vi "FindClusterCtlRefs.vi"(8 "error in (no error)":errorcluster, 10 "CLT Ref Array":refnum<vi>[](array[refnum]), 11 "CTL Name Array":string[](array[string])) -> (0 "error out":errorcluster, 2 "Cluster CTL Array":refnum<vi>[](array[refnum]), 3 "Cluster CTL Name Array":string[](array[string]))   [LabVIEW 2018, in "CtlReferences.lvlib" / "CtlReferences.lvclass"]
doc: "Get the refs of the CTLS in a Cluster.\nThis VI will also get the CTLS of any clusters inside the cluster... etc."
uses:
  CtlReferences.lvclass
  TypeDefs/ClassID_Enum.ctl
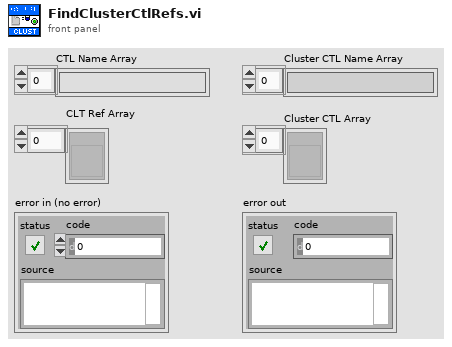
[diagram p1: front panel]
types:
  T1 = typedef "CtlReferences.lvlib/CtlReferences.lvclass/ClassID_Enum.ctl" = enum32{"0 <undefined>", "1 <undefined>", "2 <undefined>", "Generic", "Decoration", "Text", "Control", "ColorBox", "Boolean", "RefNum", "Variant", "Path", "ListBox", "Table", "Array", "Picture", "ActiveXContainer", "Numeric", "Digital", "NamedNumeric", "ColorRamp", "Slide", "GraphOrChart", "WaveformChart", "WaveformGraph", "IntensityChart", "IntensityGraph", "String", "IOName", "ComboBox", "Cluster", "Panel", "Knob", "NumWithScale", "Ring", "Enum", "GObject", "Plot", "Cursor", "NumericText", "Scale", "ColorScale", "GraphScale", "ColorGraphScale", "TypedRefNum", "OldKnobScale", "MCListbox", "MeasureData", "BVTag", "DAQName", "VISAName", "IVIName", "SlideScale", "TabControl", "Page", "TabArrayTabControl", "ConPane"}
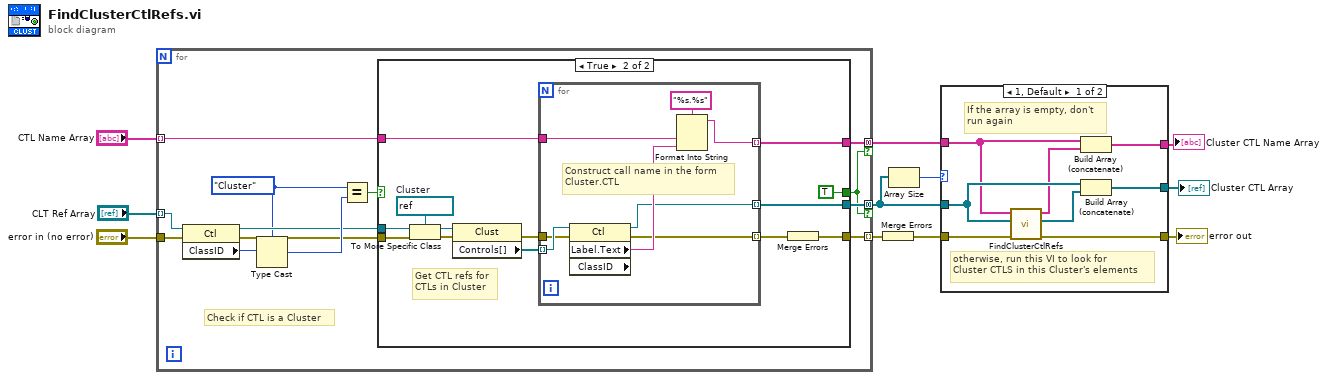
[diagram p0: block diagram]
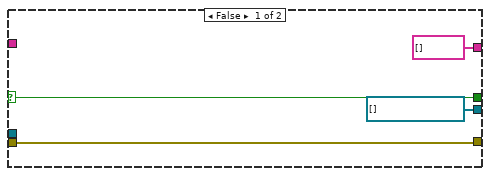
[diagram p2: hidden frame]
diagram:
  n1 = for {
    tunnel: "error in (no error)" -> [w18]
    tunnel: "CTL Name Array" -> [w23] mode=indexing
    tunnel: [w22] -> w1 mode=concatenating if=w19
    tunnel: [w21] -> w11 mode=indexing
    tunnel: [w20] -> w5 mode=concatenating if=w19
    tunnel: "CLT Ref Array" -> [w17] mode=indexing
    w12 = ClassID_Enum."Cluster" ("ClassID Name")
    # "Check if CTL is a Cluster"
    n2 = property class="Ctl"(reference=w17, error in=w18) -> (reference out=w14:refnum<vi>, error out=w13:errorcluster, "ClassID"=w16:u32)
    n3 = Type Cast(type=w12, x=w16) -> (*(type *) &x=w15:T1)
    n4 = Equal?(x=w12, y=w15) -> (x = y?=w24:bool)
    n5 = case shown="True" w24 {
      selector: w24 -> [w27 _]
      tunnel: w13 -> [w28 w41]
      tunnel: w14 -> [_ w29]
      tunnel: w23 -> [_ w35]
      tunnel: [refnum<vi>[] [] w32] -> w22
      tunnel: [w28 w33] -> w21
      tunnel: [string[] [] w31] -> w20
      tunnel: [w27 TRUE] -> w19
      frame False {
      }
      frame True {
        w40 = refnum<vi> refnum  # Cluster
        # "Get CTL refs for\nCTLs in Cluster"
        n6 = To More Specific Class(target class=w40, reference=w29, error in=w41) -> (specific class reference=w39:refnum<vi>, error out=w38:errorcluster)
        n7 = property class="Clust"(reference=w39, error in=w38) -> (error out=w36:errorcluster, "Controls[]"=w37:refnum<vi>[])  [unwired: 1 out]
        n8 = for {
          tunnel: w37 -> [w49] mode=indexing
          tunnel: w36 -> [w48]
          tunnel: w35 -> [w43]
          tunnel: [w42] -> w32 mode=indexing
          tunnel: [w45] -> w34 mode=indexing
          tunnel: [w44] -> w31 mode=indexing
          # "Construct call name in the form\nCluster.CTL"
          n9 = property class="Ctl" props=["Label", "Text", "ClassID"](reference=w49, error in=w48) -> (reference out=w42:refnum<vi>, error out=w45:errorcluster, "Label.Text"=w46:string)  [unwired: 1 out]
          n10 = Format Into String(format string="%s.%s", w43, w46) -> (resulting string=w44:string)  [unwired: 2 in, 1 out]
        }
        n11 = Merge Errors(w34) -> (w33:errorcluster)
      }
    }
  }
  n12 = Merge Errors(w11) -> (w7:errorcluster)
  n13 = Array Size(array=w1) -> (size(s)=w2:i32)
  n14 = case shown="1, Default" w2 {
    tunnel: w7 -> [w57 w58]
    tunnel: [w56 w58] -> w6
    tunnel: w1 -> [w54 w59]
    tunnel: w5 -> [w53 w60]
    tunnel: [w51 w60] -> w4
    tunnel: [w50 w59] -> w3
    frame 1, Default {
      # "otherwise, run this VI to look for\nCluster CTLS in this Cluster's elements"
      # "If the array is empty, don't\nrun again"
      n15 = call "FindClusterCtlRefs.vi"("error in (no error)"=w57, "CLT Ref Array"=w54, "CTL Name Array"=w53) -> ("error out"=w56:errorcluster, "Cluster CTL Array"=w55:refnum<vi>[], "Cluster CTL Name Array"=w52:string[])  [unwired: 6 in]
      n16 = Build Array (concatenate)(w53, w52) -> (w51:string[])
      n17 = Build Array (concatenate)(w54, w55) -> (w50:refnum<vi>[])
    }
    frame 0 {
    }
  }
  "Cluster CTL Name Array" <- w4
  "Cluster CTL Array" <- w3
  "error out" <- w6
